vi "test_scripting.vi"() -> ()   [LabVIEW 2020]
panel:
  out "save path":path
  in  "Icon file":path
  in  "Create model?":bool=TRUE
  in  "get_set":bool
  out "error out":errorcluster
  in  "Clusters":T1(array[cluster])
  in  "error in":errorcluster
  in  "Model":string
  in  "Module":string
  in  "Control Path":path=path "C:/Users/hugoc/TDF Dropbox/2_Technologies de France/1 - Services et Etudes/_Missions/HC/6 - PLAIYLAB/code/Model/Supervised/Linear_model/LinearRegressors/MultiTaskElasticNetCV/MultiTaskElasticNetCV.lvclass"
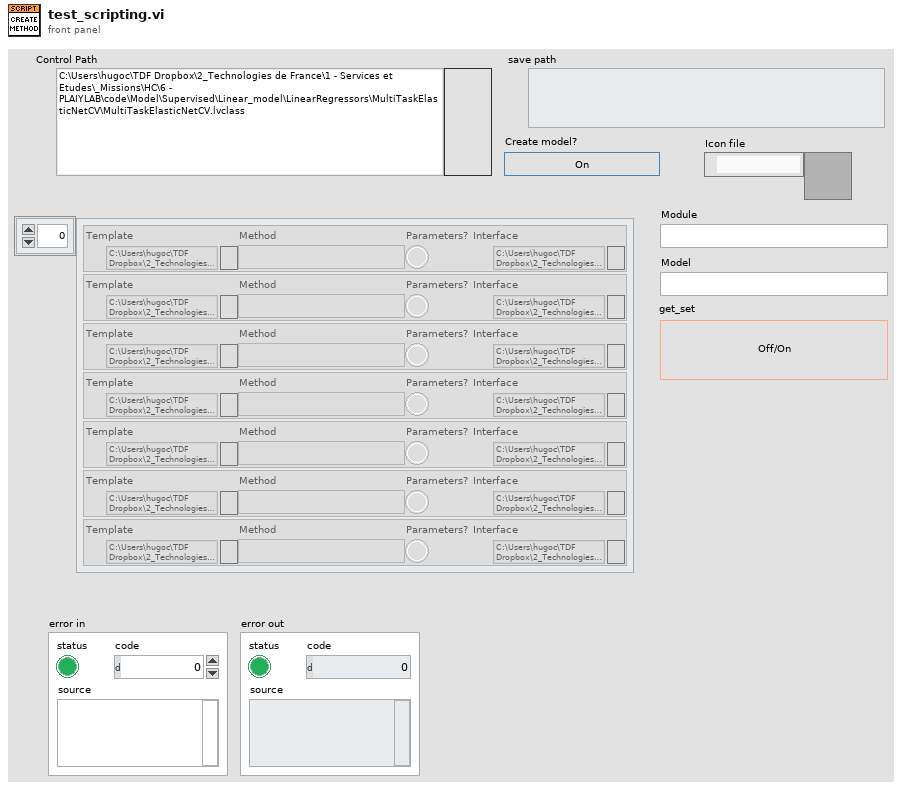
[diagram p1: front panel]
types:
  T1 = cluster{"Template":path, "Method":string, "Parameters?":bool, "Interface":path}[]
  T2 = cluster{"Template":path, "Method":string, "Parameters?":bool, "Interface":path}
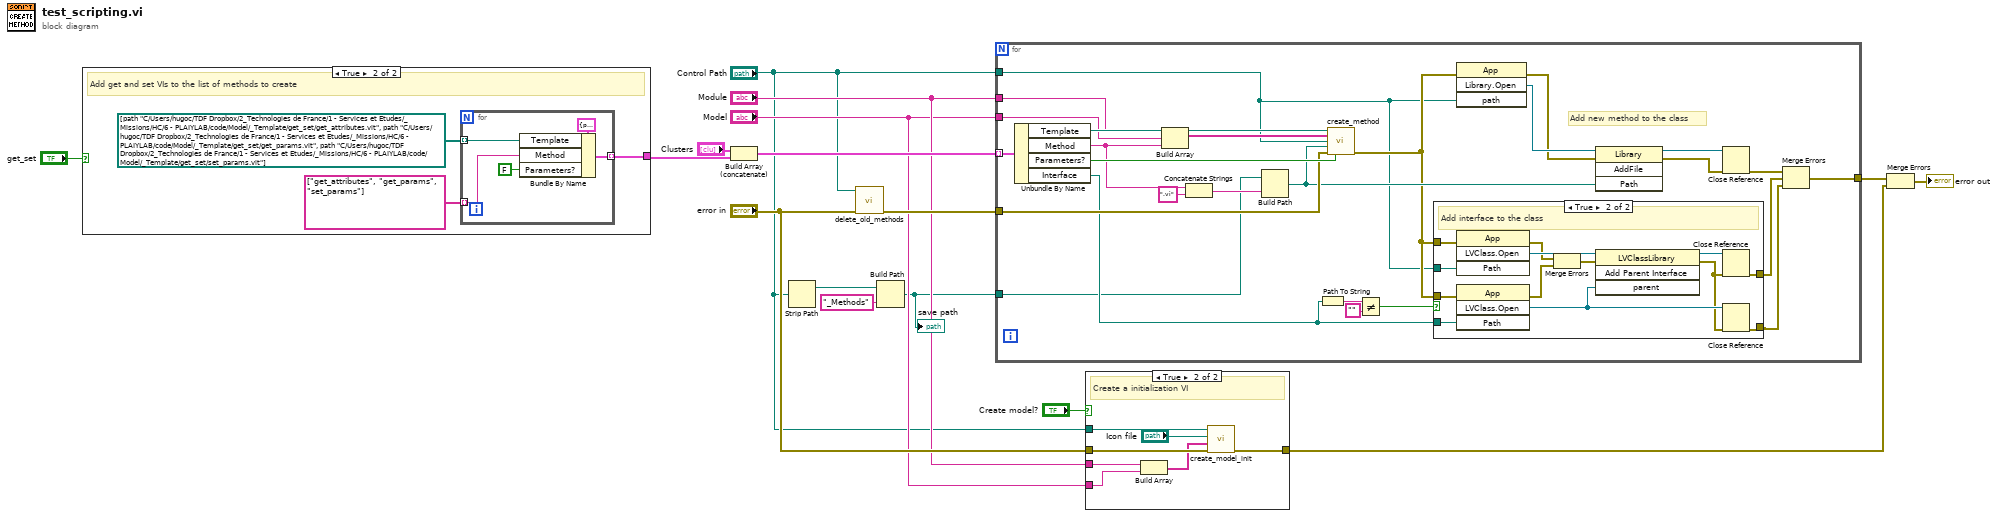
[diagram p0: block diagram]
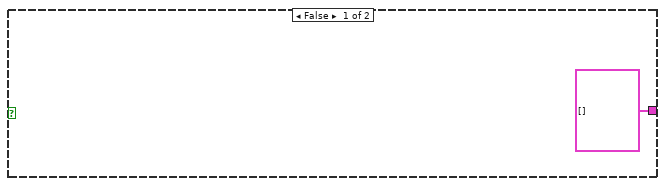
[diagram p3: hidden frame]
diagram:
  n1 = case shown="True" "get_set" {
    tunnel: [T1 [] w18] -> w14
    frame False {
    }
    frame True {
      # "Add get and set VIs to the list of methods to create"
      n2 = for {
        tunnel: path[] [path "C:/Users/hugoc/TDF Dropbox/2_Technologies de France/1 - Services et Etudes/_Missions/HC/6 - PLAIYLAB/code/Model/_Template/get_set/get_attributes.vit", path "C:/Users/hugoc/TDF Dropbox/2_Technologies de France/1 - Services et Etudes/_Missions/HC/6 - PLAIYLAB/code/Model/_Template/get_set/get_params.vit", path "C:/Users/hugoc/TDF Dropbox/2_Technologies de France/1 - Services et Etudes/_Missions/HC/6 - PLAIYLAB/code/Model/_Template/get_set/set_params.vit"] -> [w25] mode=indexing
        tunnel: string[] ["get_attributes", "get_params", "set_params"] -> [w24] mode=indexing
        tunnel: [w22] -> w18 mode=indexing
        n3 = Bundle By Name(cluster=T2 {"Template"=path "", "Method"="", "Parameters?"=FALSE, "Interface"=path ""} ("Methods"), "Template"=w25, "Method"=w24, "Parameters?"=FALSE) -> (w22:T2)
      }
    }
  }
  n4 = Build Array (concatenate)("Clusters", w14) -> (w16:T1)
  n5 = Strip Path(path="Control Path") -> (stripped path=w4:path)  [unwired: 1 out]
  n6 = call "delete_old_methods.vi"("error in (no error)"="error in", "Path"="Control Path") -> ("error out"=w7:errorcluster)  [unwired: 9 in]
  n7 = Build Path(base path=w4, name or relative path="_Methods") -> (appended path=w1:path)
  "save path" <- w1
  n8 = for {
    tunnel: "Module" -> [w47]
    tunnel: "Model" -> [w46]
    tunnel: w7 -> [w43]
    tunnel: w16 -> [w50] mode=indexing
    tunnel: [w36] -> w11
    tunnel: w1 -> [w29]
    tunnel: "Control Path" -> [w28]
    # "Add new method to the class"
    n9 = Unbundle By Name(w50) -> ("Template"=w48:path, "Method"=w30:string, "Parameters?"=w44:bool, "Interface"=w35:path)
    n10 = Build Array(w47, w46, w30) -> (w45:string[])
    n11 = Concatenate Strings(w30, ".vi" ("string")) -> (w49:string)
    n12 = Build Path(base path=w29, name or relative path=w49) -> (appended path=w41:path)
    n13 = Path To String(path=w35) -> (string=w34:string)
    n14 = call "create_method.vi"("template_path"=w48, "ModuleModelFunction"=w45, "Control Path"=w28, "Path to Saved File"=w41, "error in (no error)"=w43, "Parameters?"=w44) -> ("error out"=w31:errorcluster)  [unwired: 9 in]
    n15 = Not Equal?(x=w34, y="") -> (x != y?=w32:bool)
    n16 = case shown="True" w32 {
      tunnel: w28 -> [_ w66]
      tunnel: w31 -> [w53 w60]
      tunnel: w35 -> [_ w64]
      tunnel: w31 -> [w52 w59]
      tunnel: [w53 w55] -> w27
      tunnel: [w52 w54] -> w26
      frame False {
      }
      frame True {
        # "Add interface to the class"
        n17 = invoke class="App" method="LVClass.Open"(error in=w60, "Path"=w66) -> (error out=w63:errorcluster, "LVClass.Open"=w65:refnum<vi>)  [unwired: 2 in, 2 out]
        n18 = invoke class="App" method="LVClass.Open"(error in=w59, "Path"=w64) -> (error out=w62:errorcluster, "LVClass.Open"=w57:refnum<vi>)  [unwired: 2 in, 2 out]
        n19 = Merge Errors(w63, w62) -> (w61:errorcluster)
        n20 = invoke class="LVClassLibrary" method="Add Parent Interface"(reference=w65, error in=w61, "parent"=w57) -> (reference out=w58:refnum<vi>, error out=w56:errorcluster)  [unwired: 1 in, 2 out]
        n21 = Close Reference(reference=w58, error in (no error)=w56) -> (error out=w55:errorcluster)
        n22 = Close Reference(reference=w57, error in (no error)=w56) -> (error out=w54:errorcluster)
      }
    }
    n23 = invoke class="App" method="Library.Open"(error in=w31, "path"=w28) -> (error out=w40:errorcluster, "Open Library"=w42:refnum<vi>)  [unwired: 2 in, 2 out]
    n24 = invoke class="Library" method="AddFile"(reference=w42, error in=w40, "Path"=w41) -> (reference out=w39:refnum<vi>, error out=w38:errorcluster)  [unwired: 1 in, 2 out]
    n25 = Close Reference(reference=w39, error in (no error)=w38) -> (error out=w37:errorcluster)
    n26 = Merge Errors(w37, w27, w26) -> (w36:errorcluster)
  }
  n27 = case shown="True" "Create model?" {
    tunnel: "Control Path" -> [_ w69]
    tunnel: [w67 w68] -> w10
    tunnel: "error in" -> [w67 w74]
    tunnel: "Module" -> [_ w72]
    tunnel: "Model" -> [_ w71]
    frame False {
    }
    frame True {
      # "Create a initialization VI"
      n28 = Build Array(w72, w71) -> (w70:string[])
      n29 = call "create_model_init.vi"("error in (no error)"=w74, "ModuleModel"=w70, "Icon file"="Icon file", "Control Path"=w69) -> ("error out"=w68:errorcluster)  [unwired: 7 in]
    }
  }
  n30 = Merge Errors(w11, w10) -> (→"error out":errorcluster)
